vi "RB2 create post string.vi"(0 "White dot\nLocation":T1(array[cluster])) -> (1 "Num Posts":i32, 2 "Post String":string)   [LabVIEW 2012]
doc: "This VI takes in an array of white post locations and creates a string with their locations."
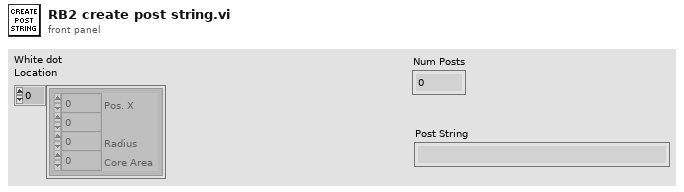
[diagram p1: front panel]
types:
  T1 = cluster{"Pos. X":i32, "Pos. Y":i32, "Radius":i32, "Core Area":i32}[]
  T2 = cluster{"Pos. X":i32, "Pos. Y":i32, "Radius":i32, "Core Area":i32}
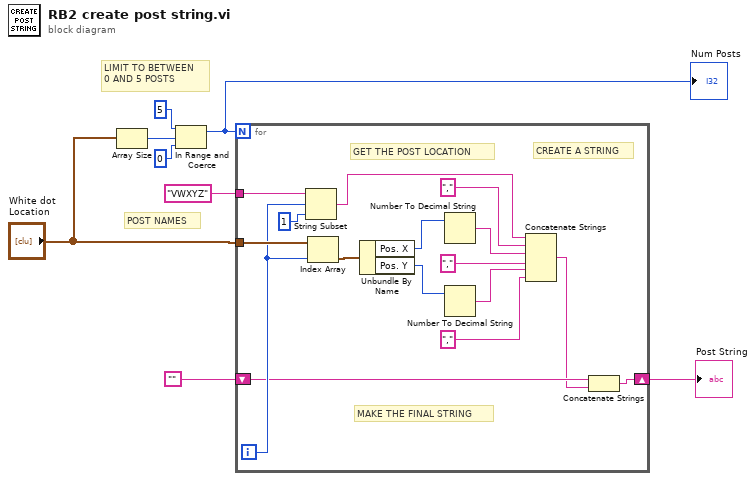
[diagram p0: block diagram]
diagram:
  # "POST NAMES"
  # "LIMIT TO BETWEEN\n0 AND 5 POSTS"
  n1 = Array Size(array="White dot\nLocation") -> (size(s)=w6:i32)
  n2 = In Range and Coerce(upper limit=5, x=w6, lower limit=0) -> (coerced(x)=w3:i32)  [unwired: 1 out]
  "Num Posts" <- w3
  n3 = for {
    N: w3 -> [_]
    tunnel: "White dot\nLocation" -> [w23]
    tunnel: "VWXYZ" -> [w18]
    shift-right: [w10] -> w1
    shift-left: "" -> [w11]
    i -> [w17]
    # "CREATE A STRING"
    # "GET THE POST LOCATION"
    # "MAKE THE FINAL STRING"
    n4 = String Subset(string=w18, offset (0)=w17, length (rest)=1 ("length (rest)")) -> (substring=w15:string)
    n5 = Index Array(array=w23, index=w17) -> (element=w24:T2)
    n6 = Unbundle By Name(w24) -> ("Pos. X"=w13:i32, "Pos. Y"=w12:i32)
    n7 = Number To Decimal String(number=w13) -> (decimal integer string=w19:string)  [unwired: 1 in]
    n8 = Number To Decimal String(number=w12) -> (decimal integer string=w21:string)  [unwired: 1 in]
    n9 = Concatenate Strings(w15, ",", w19, ",", w21, ",") -> (w9:string)
    n10 = Concatenate Strings(w11, w9) -> (w10:string)
  }
  "Post String" <- w1
